vi "get both TA and MQT.vi"(0 "path in":path, 5 "Points":i32, 7 "Start current":dbl, 9 "Step":dbl, 11 "error in (no error)":errorcluster) -> (4 "path out":path, 6 "I":dbl[](array[numeric]), 8 "TA":dbl[](array[numeric]), 10 "MQT":dbl[](array[numeric]), 15 "error out":errorcluster)   [LabVIEW 2023]
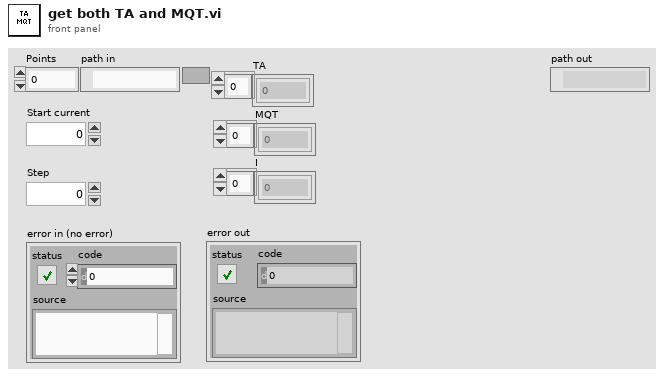
[diagram p1: front panel]
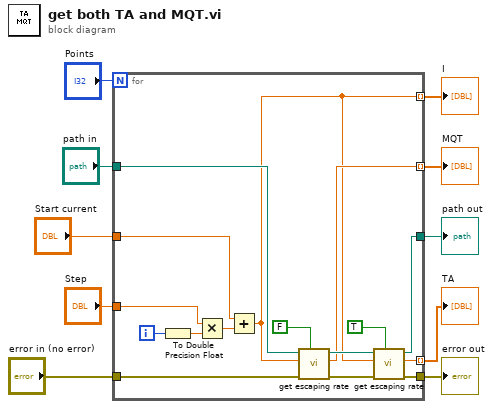
[diagram p0: block diagram]
diagram:
  n1 = for {
    N: "Points" -> [_]
    tunnel: "Start current" -> [w26]
    tunnel: "Step" -> [w24]
    tunnel: "error in (no error)" -> [w19]
    tunnel: [w17] -> w6
    tunnel: [w16] -> w5 mode=indexing
    tunnel: [w13] -> w4 mode=indexing
    tunnel: [w12] -> w3 mode=indexing
    tunnel: "path in" -> [w14]
    tunnel: [w11] -> w1
    i -> [w25]
    n2 = To Double Precision Float(number=w25) -> (double precision float=w23:dbl)
    n3 = Multiply(x=w24, y=w23) -> (x*y=w22:dbl)
    n4 = Add(x=w26, y=w22) -> (x+y=w12:dbl)
    n5 = call "get escaping rate.vi"("TA or MQT"=FALSE, "error in (no error)"=w19, "current"=w12, "path in"=w14) -> ("error out"=w18:errorcluster, "rate"=w13:dbl, "path out"=w15:path)  [unwired: 5 in]
    n6 = call "get escaping rate.vi"("TA or MQT"=TRUE, "error in (no error)"=w18, "current"=w12, "path in"=w15) -> ("error out"=w17:errorcluster, "rate"=w16:dbl, "path out"=w11:path)  [unwired: 5 in]
  }
  "error out" <- w6
  "TA" <- w5
  "MQT" <- w4
  "I" <- w3
  "path out" <- w1
